vi "Using MouseDown Event Callback to Change Front Panel Functionality.vi"() -> ()   [LabVIEW 2017]
panel:
  in  "Listbox 2":i32(listbox)
  in  "stop":bool
  in  "Listbox":i32(listbox)
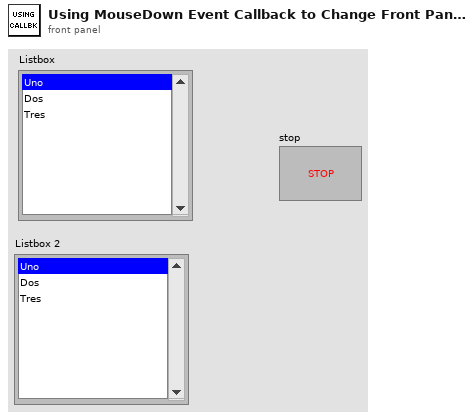
[diagram p1: front panel]
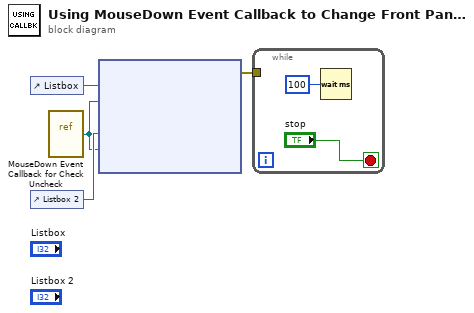
[diagram p0: block diagram]
diagram:
  n1 = control-ref of="Listbox"() -> (w4:refnum<vi>)
  n2 = control-ref of="Listbox 2"() -> (w3:refnum<vi>)
  n3 = vi-ref "MouseDown Event Callback for Check Uncheck.vi"() -> ("vi reference"=w2:refnum<vi>)
  n4 = node(w4, w2, w3, w2) -> (w1:errorcluster)  [unwired: 4 in, 1 out]
  n5 = while {
    tunnel: w1 -> [_]
    stop <- "stop" stop-if-true
    n6 = Wait (ms)(milliseconds to wait=u32 100) -> ()  [unwired: 1 out]
  }
